vi "Untitled 1.vi"() -> ()   [LabVIEW 2020]
uses:
  <vilib>/Instr/_visa.llb/VISA Configure Serial Port (Instr).vi
panel:
  in  "millisecond timer value":u32
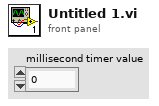
[diagram p1: front panel]
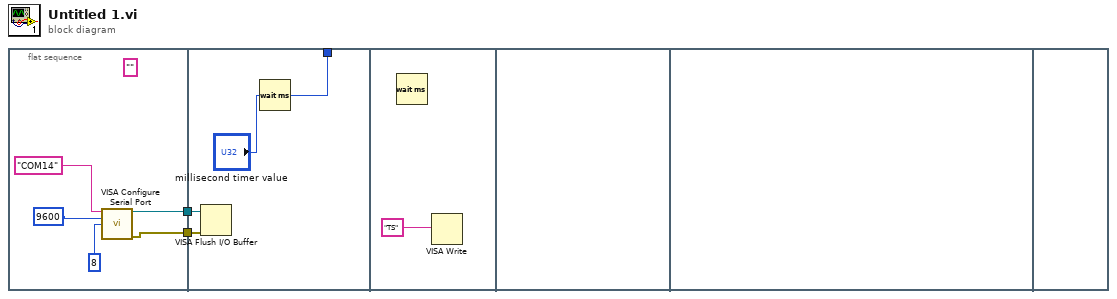
[diagram p0: block diagram]
diagram:
  n1 = flat-sequence {
    tunnel: [w4] -> w2
    tunnel: [w3] -> w1
    tunnel: w2 -> [w11]
    tunnel: w1 -> [w10]
    tunnel: [w8] -> _
    frame #0 {
      (unwired) ""
      n2 = call-poly "VISA Configure Serial Port"("VISA resource name"="COM14", "baud rate (9600)"=9600, "data bits (8)"=8) -> ("VISA resource name out"=w3:refnum<visa-resource-name>, "error out"=w4:errorcluster)  [unwired: 11 in]
    }
    frame #1 {
      n3 = VISA Flush I/O Buffer(VISA resource name=w10, error in (no error)=w11) -> ()  [unwired: 1 in, 2 out]
      n4 = Wait (ms)(milliseconds to wait="millisecond timer value") -> (millisecond timer value=w8:u32)
    }
    frame #2 {
      n5 = Wait (ms)() -> ()  [unwired: 1 in, 1 out]
      n6 = VISA Write(write buffer="TS") -> ()  [unwired: 2 in, 3 out]
    }
    frame #3 {
    }
    frame #4 {
    }
    frame #5 {
    }
  }
